vi "Select ECUMC Item.vi"(6 "NIVS.System Definition Root":refnum<k24>, 8 "error in (no error)":errorcluster, 9 "Item Type":T1=enum."Measurement", 11 "Link In":T2) -> (0 "error out":errorcluster, 1 "Canceled?":bool, 3 "Link Out":T2)   [LabVIEW 2011]
uses:
  <vilib>/ECUMC/NIVS/Support Files.llb/Comment Property.ctl
  <vilib>/ECUMC/NIVS/Support Files.llb/Address Property.ctl
  <vilib>/ECUMC/NIVS/Support Files.llb/Extension Property.ctl
  <vilib>/ECUMC/NIVS/Support Files.llb/Unit Property.ctl
  NationalInstruments.VeriStand.SystemStorage
  Controls/ECUMC Item.ctl
  <vilib>/ECUMC/NIVS/Support Files.llb/Item Type.ctl
  <vilib>/ECUMC/NIVS/Support Files.llb/Get Single Char Properties (TCP).vi
  <vilib>/ECUMC/NIVS/Support Files.llb/Get Single Meas Properties (TCP).vi
  <userlib>/_OpenG.lib/array/array.llb/Filter 1D Array__ogtk.vi
  <userlib>/_OpenG.lib/array/array.llb/Filter 1D Array with Scalar (String)__ogtk.vi
  <userlib>/_OpenG.lib/string/string.llb/String to 1D Array__ogtk.vi
  <vilib>/dlg_ctls.llb/Space Constant.vi
  NationalInstruments.VeriStand.SystemDefinitionAPI
  <vilib>/ECUMC/NIVS/Support Files.llb/XCP and CCP Master Custom Device.lvlib
  <vilib>/ECUMC/NIVS/XCPCCP Add-On Execution API.lvlib
panel:
  in  "Target":u16(ring) items=["FirstController"]
  in  "Cancel":bool
  in  "OK":bool
  out "Unit":T3
  out "Extension":T4
  out "Address":T5 format="%x"
  out "Comment":T6
  in  "Show results:":enum32{"Radio Selection 2", "Radio Selection 1"}(radio)
  in  "CaseSens":bool
  in  "Search":string
  in  "ItemList":i32(listbox) caption="Available Items in Database"
  in  "CD":u16(ring) caption="Custom Device" items=["XCP and CCP Master"]
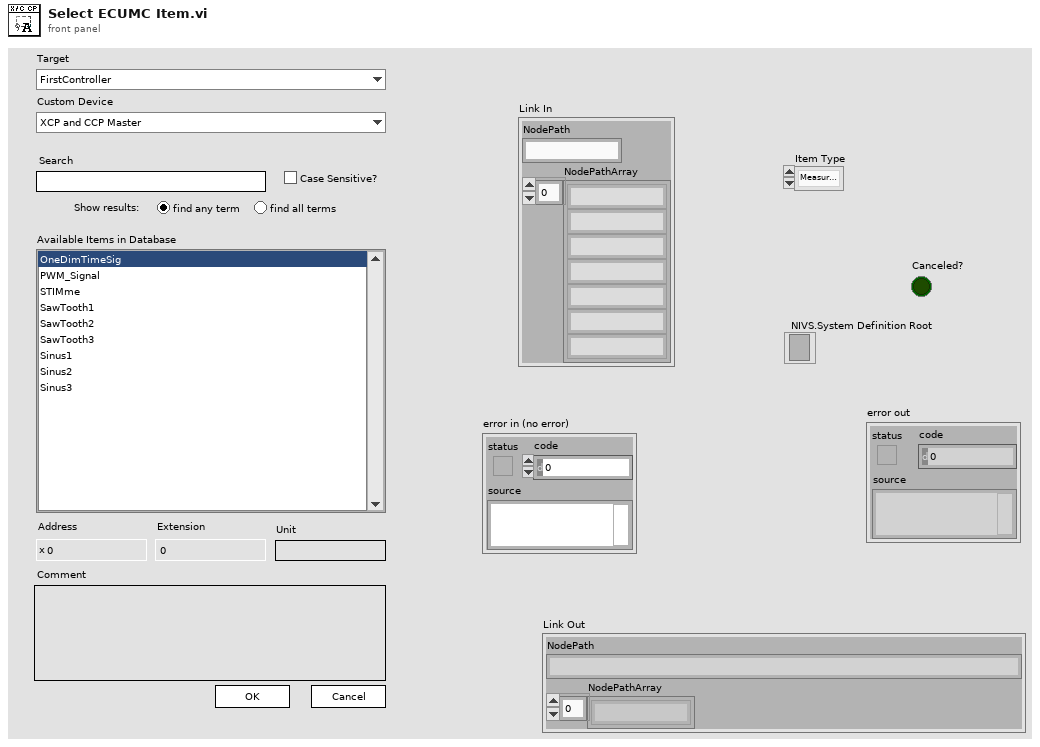
[diagram p1: front panel]
types:
  T1 = typedef "XCP and CCP Master Custom Device.lvlib/Item Type.ctl" = enum16{"Scalar Characteristic", "Curve Characteristic", "Field Characteristic", "Measurement"}
  T2 = typedef "ECUMC Item.ctl" = cluster{"NodePath":string, "NodePathArray":string[]}
  T3 = typedef "XCP and CCP Master Custom Device.lvlib/Unit Property.ctl" = string
  T4 = typedef "XCP and CCP Master Custom Device.lvlib/Extension Property.ctl" = u8
  T5 = typedef "XCP and CCP Master Custom Device.lvlib/Address Property.ctl" = u32
  T6 = typedef "XCP and CCP Master Custom Device.lvlib/Comment Property.ctl" = string
  T7 = typedef "XCP and CCP Master Custom Device.lvlib/Item Properties.ctl" = cluster{"Common":cluster{"Address":T5, "Extension":T4, "Data Type":T8, "Byte Order":T9, "Maximum":T10, "Minimum":T11, "Read Only?":T12, "Unit":T3, "Comment":T6}, "Char Specific":cluster{"X Dimension":T13, "Y Dimension":T14, "char x axis":dbl[], "char y axis":dbl[], "char sizes":u32[]}, "Meas Specific":cluster{"Virtual?":T15}}
  T8 = typedef "XCP and CCP Master Custom Device.lvlib/Data Type Property.ctl" = enum16{"UBYTE", "SBYTE", "UWORD", "SWORD", "ULONG", "SLONG", "FLOAT32_IEEE", "FLOAT64_IEEE"}
  T9 = typedef "XCP and CCP Master Custom Device.lvlib/Byte Order Property.ctl" = enum16{"Intel", "Motorola"}
  T10 = typedef "XCP and CCP Master Custom Device.lvlib/Maximum Property.ctl" = dbl
  T11 = typedef "XCP and CCP Master Custom Device.lvlib/Minimum Property.ctl" = dbl
  T12 = typedef "XCP and CCP Master Custom Device.lvlib/Read Only Property.ctl" = bool
  T13 = typedef "XCP and CCP Master Custom Device.lvlib/X Dimension Property.ctl" = u32
  T14 = typedef "XCP and CCP Master Custom Device.lvlib/Y Dimension Property.ctl" = u32
  T15 = typedef "XCP and CCP Master Custom Device.lvlib/Is Virtual Property.ctl" = bool
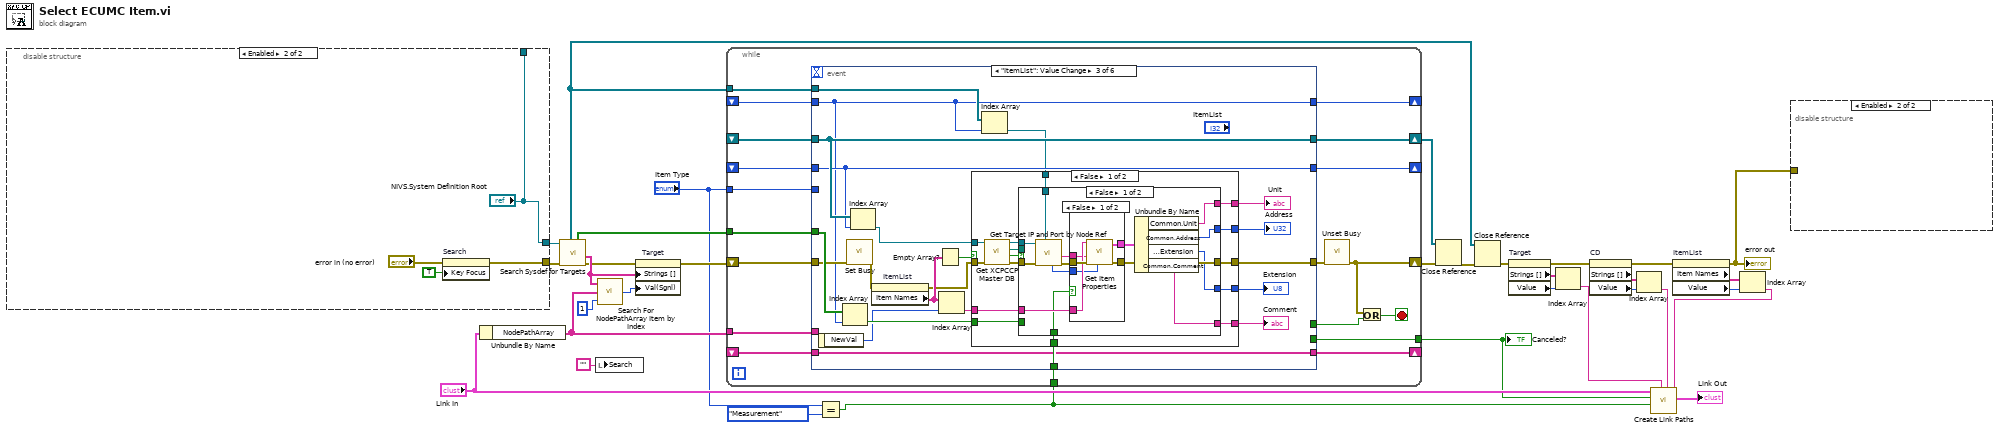
[diagram p0: block diagram]
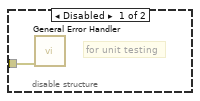
[diagram p2: hidden frame]
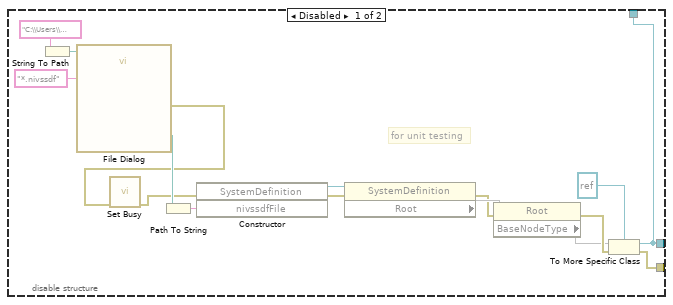
[diagram p3: hidden frame]
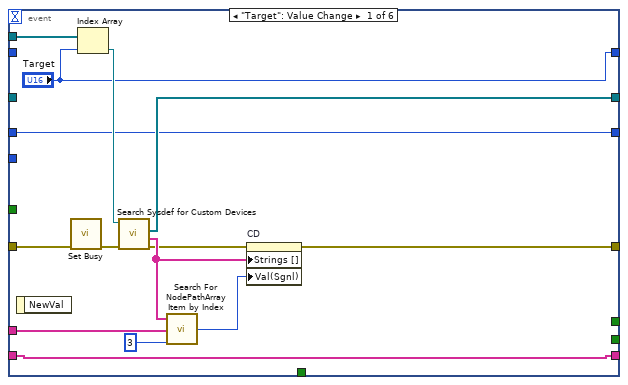
[diagram p4: hidden frame]
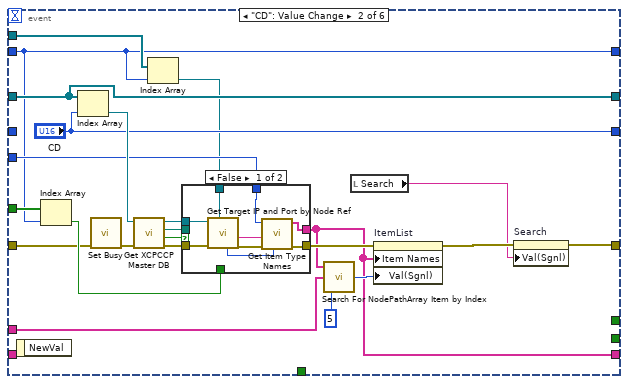
[diagram p5: hidden frame]
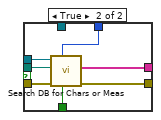
[diagram p6: hidden frame]
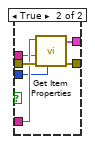
[diagram p7: hidden frame]
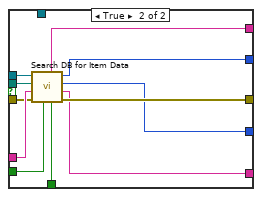
[diagram p8: hidden frame]
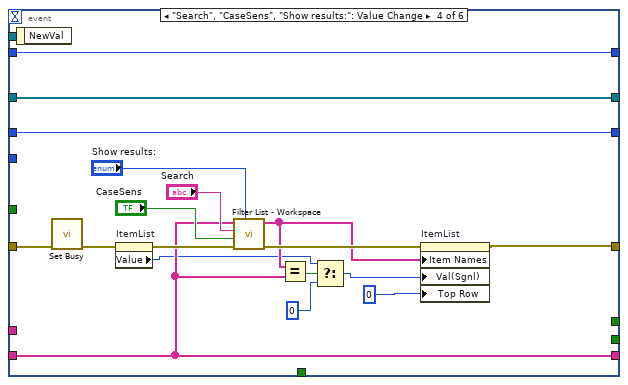
[diagram p10: hidden frame]
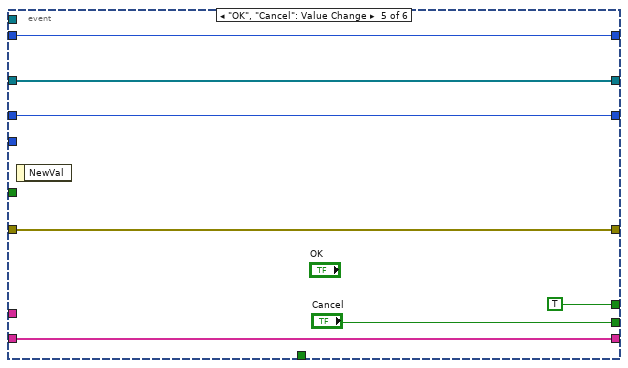
[diagram p11: hidden frame]
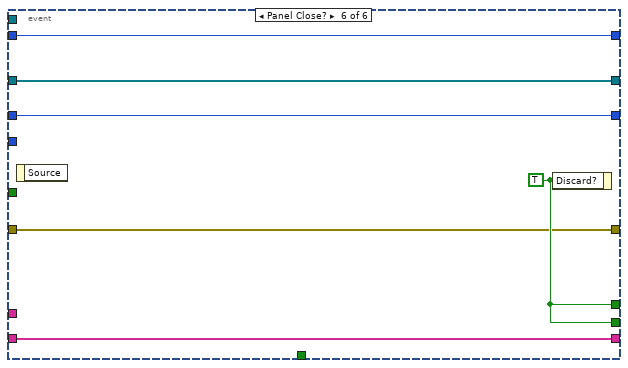
[diagram p12: hidden frame]
diagram:
  n1 = disable-structure shown="Enabled" {
    disable-tunnel: [w34 "NIVS.System Definition Root"] -> w32
    disable-tunnel: [w41 w50] -> w21
    disable-tunnel: [w34 "NIVS.System Definition Root"] -> _
    frame Disabled {
      # "for unit testing"
      n2 = String To Path(string="C:\\Users\\Public\\Documents\\National Instruments\\NI VeriStand 2010\\Projects") -> (path=w37:path)
      n3 = call "File Dialog"("start path"=w37, "pattern (all files)"="*.nivssdf") -> ("selected path"=w48:path, "error out"=w35:errorcluster)  [unwired: 10 in, 2 out]
      n4 = call <vilib>:"Set Busy.vi"("error in (no error)"=w35) -> ("error out"=w36:errorcluster)  [unwired: 9 in, 1 out]
      n5 = Path To String(path=w48) -> (string=w47:string)
      n6 = constructor class="SystemDefinition"(error in=w36, "nivssdfFile"=w47) -> (reference out=w45:refnum<k24>, error out=w46:errorcluster)  [unwired: 2 in, 2 out]
      n7 = property class="SystemDefinition"(reference=w45, error in=w46) -> (error out=w43:errorcluster, "Root"=w44)  [unwired: 1 out]
      n8 = property class="Root"(reference=w44, error in=w43) -> (error out=w42:errorcluster, "BaseNodeType"=w40)  [unwired: 1 out]
      n9 = To More Specific Class(target class=refnum<k24> refnum, reference=w40, error in=w42) -> (specific class reference=w34:refnum<k24>, error out=w41:errorcluster)
    }
    frame Enabled {
      n10 = property on="Search" class="Str"(error in="error in (no error)", "Key Focus"=TRUE) -> (error out=w50:errorcluster)  [unwired: 1 in, 1 out]
    }
  }
  n11 = Unbundle By Name("Link In") -> ("NodePathArray"=w27:string[])
  n12 = call "Search Sysdef for Targets.vi"("error in (no error)"=w21, "NIVS.System Definition Root"=w32) -> ("error out"=w22:errorcluster, "Target Names"=w29:string[], "Windows?"=w31:bool[], "Target Nodes"=w23:refnum<k24>[])  [unwired: 5 in, 1 out]
  n13 = local write "Search"("") -> ()
  n14 = call "Search For NodePathArray Item by Index.vi"("index of NodePathArray"=1 ("index"), "NodePathArray"=w27, "Items to search"=w29) -> ("result"=w28:i32)
  n15 = property on="Target" class="Ring (strict)"(error in=w22, "Strings []"=w29, "Val(Sgnl)"=w28) -> (error out=w5:errorcluster)  [unwired: 1 in, 1 out]
  n16 = Equal?(x="Item Type", y=Item_Type."Measurement") -> (x = y?=w2:bool)
  n17 = while {
    shift-right: [w54] -> w26
    shift-left: w5 -> [w72]
    tunnel: w31 -> [w70]
    tunnel: w27 -> [w69]
    tunnel: w23 -> [w68]
    tunnel: [w66] -> w19
    shift-right: [w65] -> w25
    shift-left: _ -> [w64]
    shift-right: [w63] -> _
    shift-left: _ -> [w62]
    shift-right: [w61] -> _
    shift-left: _ -> [w60]
    tunnel: "Item Type" -> [w59]
    tunnel: w2 -> [w58]
    shift-right: [w57] -> _
    shift-left: _ -> [w56]
    stop <- w71 stop-if-true
    n18 = event shown="[2] \"ItemList\": Value Change" {
      selector: _ -> [_ _ _ _ _ _]
      dyn-events: _ -> [_ _ _ _ _ _]
      timeout: _ -> [_ _ _ _ _ _]
      tunnel: w72 -> [w79 w101 w141 w203 w225 w226]
      tunnel: w70 -> [_ w103 w144 _ _ _]
      tunnel: w69 -> [w82 w106 _ _ _ _]
      tunnel: w68 -> [w86 w89 w137 _ _ _]
      tunnel: [_ _ _ _ TRUE w230] -> w67
      tunnel: [w73 w90 w126 w201 w225 w226] -> w55
      tunnel: [_ _ _ _ "Cancel" w230] -> w66
      tunnel: w62 -> [_ w88 w136 w212 w220 w227]
      tunnel: [w84 w99 w147 w213 w222 w228] -> w65
      tunnel: w64 -> [_ w99 w147 w213 w222 w228]
      tunnel: ["Target" w88 w136 w212 w220 w227] -> w63
      tunnel: [w75 "CD" w146 w214 w221 w229] -> w61
      tunnel: w60 -> [w75 _ w146 w214 w221 w229]
      tunnel: w59 -> [_ w96 _ _ _ _]
      tunnel: w58 -> [_ _ w142 _ _ _]
      tunnel: [w74 w95 w140 w209 w219 w231] -> w57
      tunnel: w56 -> [w74 _ w140 w209 w219 w231]
      event "Target": Value Change {
        n19 = event-data() -> ()  [unwired: 1 in, 1 out]
        n20 = call <vilib>:"Set Busy.vi"("error in (no error)"=w79) -> ("error out"=w78:errorcluster)  [unwired: 9 in, 1 out]
        n21 = Index Array(array=w86, index="Target") -> (element=w85:refnum<k24>)
        n22 = call "Search Sysdef for Custom Devices.vi"("error in (no error)"=w78, "Target Node"=w85) -> ("error out"=w77:errorcluster, "Custom Device Names"=w83:string[], "Custom Device Nodes"=w84:refnum<k24>[])  [unwired: 6 in, 1 out]
        n23 = call "Search For NodePathArray Item by Index.vi"("index of NodePathArray"=3 ("index"), "NodePathArray"=w82, "Items to search"=w83) -> ("result"=w80:i32)
        n24 = property on="CD" class="Ring (strict)"(error in=w77, "Strings []"=w83, "Val(Sgnl)"=w80) -> (error out=w73:errorcluster)  [unwired: 1 in, 1 out]
      }
      event "CD": Value Change {
        n25 = event-data() -> ()  [unwired: 1 in, 1 out]
        n26 = Index Array(array=w103, index=w88) -> (element=w102:bool)
        n27 = Index Array(array=w99, index="CD") -> (element=w109:refnum<k24>)
        n28 = call <vilib>:"Set Busy.vi"("error in (no error)"=w101) -> ("error out"=w100:errorcluster)  [unwired: 9 in, 1 out]
        n29 = call "Get XCPCCP Master DB.vi"("error in (no error)"=w100, "Custom Device Node in"=w109) -> ("error out"=w108:errorcluster, "file or folder exists?"=w92:bool, "DB Path"=w91:path, "Custom Device Node out"=w107:refnum<k24>)  [unwired: 6 in]
        n30 = Index Array(array=w89, index=w88) -> (element=w87:refnum<k24>)
        n31 = case shown="False" w92 {
          tunnel: w108 -> [w115 w125]
          tunnel: w91 -> [_ w120]
          tunnel: w107 -> [w114 w123]
          tunnel: [w117 w121] -> w95
          tunnel: [w118 w124] -> w104
          tunnel: w96 -> [w116 w122]
          tunnel: w102 -> [_ w119]
          tunnel: w87 -> [w113 _]
          frame False {
            n32 = call "Get Target IP and Port by Node Ref.vi"("Target Node In"=w113, "error in (no error)"=w115, "Custom Device Node in"=w114) -> ("error out"=w111:errorcluster, "IP"=w110:string, "Port"=w112:u16)  [unwired: 6 in]
            n33 = call <vilib>:"Get Item Type Names.vi"("Port"=w112, "error in (no error)"=w111, "IP or DNS Name"=w110, "Item Type"=w116) -> ("error out"=w118:errorcluster, "Names"=w117:string[])  [unwired: 6 in]
          }
          frame True {
            n34 = call "Search DB for Chars or Meas.vi"("Windows? (F)"=w119, "Item Type"=w122, "error in (no error)"=w125, "DB Path"=w120, "Custom Device Node in"=w123) -> ("error out"=w124:errorcluster, "Chans"=w121:string[])  [unwired: 4 in, 1 out]
          }
        }
        n35 = call "Search For NodePathArray Item by Index.vi"("index of NodePathArray"=5, "NodePathArray"=w106, "Items to search"=w95) -> ("result"=w98:i32)
        n36 = local read "Search"() -> (w93:string)
        n37 = property on="ItemList" class="LstBox (strict)"(error in=w104, "Item Names"=w95, "Val(Sgnl)"=w98) -> (error out=w94:errorcluster)  [unwired: 1 in, 1 out]
        n38 = property on="Search" class="Str"(error in=w94, "Val(Sgnl)"=w93) -> (error out=w90:errorcluster)  [unwired: 1 in, 1 out]
      }
      event "ItemList": Value Change {
        n39 = event-data() -> ("NewVal"=w139:i32)  [unwired: 1 in]
        n40 = Index Array(array=w144, index=w136) -> (element=w143:bool)
        n41 = call <vilib>:"Set Busy.vi"("error in (no error)"=w141) -> ("error out"=w130:errorcluster)  [unwired: 9 in, 1 out]
        n42 = Index Array(array=w147, index=w146) -> (element=w145:refnum<k24>)
        n43 = property on="ItemList" class="LstBox (strict)"(error in=w130) -> (error out=w128:errorcluster, "Item Names"=w129:string[])  [unwired: 1 in, 1 out]
        n44 = Empty Array?(array=w129) -> (empty?=w127:bool)
        n45 = Index Array(array=w129, index=w139) -> (element=w138:string)
        n46 = Index Array(array=w137, index=w136) -> (element=w135:refnum<k24>)
        n47 = case shown="False" w127 {
          tunnel: w145 -> [w162 _]
          tunnel: w143 -> [w160 _]
          tunnel: w142 -> [w157 _]
          tunnel: [w156 w200] -> w126
          tunnel: w138 -> [w155 _]
          tunnel: w135 -> [w154 _]
          tunnel: [w153 _] -> w134
          tunnel: [w152 _] -> w133
          tunnel: [w151 _] -> w132
          tunnel: [w150 _] -> w131
          tunnel: w128 -> [w149 w200]
          frame False {
            n48 = call "Get XCPCCP Master DB.vi"("error in (no error)"=w149, "Custom Device Node in"=w162) -> ("error out"=w148:errorcluster, "file or folder exists?"=w161:bool, "DB Path"=w158:path, "Custom Device Node out"=w159:refnum<k24>)  [unwired: 6 in]
            n49 = case shown="False" w161 {
              tunnel: w160 -> [_ w199]
              tunnel: w159 -> [w173 w198]
              tunnel: w158 -> [_ w197]
              tunnel: w148 -> [w175 w193]
              tunnel: w157 -> [w168 w196]
              tunnel: [w169 w195] -> w156
              tunnel: w155 -> [w176 w194]
              tunnel: w154 -> [w172 _]
              tunnel: [w163 w192] -> w153
              tunnel: [w164 w191] -> w152
              tunnel: [w165 w190] -> w151
              tunnel: [w166 w189] -> w150
              frame False {
                n50 = call "Get Target IP and Port by Node Ref.vi"("Target Node In"=w172, "error in (no error)"=w175, "Custom Device Node in"=w173) -> ("error out"=w174:errorcluster, "IP"=w170:string, "Port"=w171:u16)  [unwired: 6 in]
                n51 = case shown="False" w168 {
                  tunnel: w174 -> [w182 w188]
                  tunnel: w176 -> [w181 w187]
                  tunnel: w171 -> [w180 w186]
                  tunnel: w170 -> [w179 w185]
                  tunnel: [w178 w184] -> w169
                  tunnel: [w177 w183] -> w167
                  frame False {
                    n52 = call-poly <vilib>:"Get Item Properties.vi"("Port"=w180, "error in (no error)"=w182, "IP or DNS Name"=w179, "Characteristic"=w181) -> ("error out"=w178:errorcluster, "Properties"=w177:T7)  [unwired: 6 in]
                  }
                  frame True {
                    n53 = call-poly <vilib>:"Get Item Properties.vi"("Port"=w186, "error in (no error)"=w188, "IP or DNS Name"=w185, "Measurement"=w187) -> ("error out"=w184:errorcluster, "Properties"=w183:T7)  [unwired: 6 in]
                  }
                }
                n54 = Unbundle By Name(w167) -> ("Common.Unit"=w166:T3, "Common.Address"=w165:T5, "Common.Extension"=w164:T4, "Common.Comment"=w163:T6)
              }
              frame True {
                n55 = call "Search DB for Item Data.vi"("Measurement? (F)"=w196, "Windows? (F)"=w199, "error in (no error)"=w193, "Item Name"=w194, "DB Path"=w197, "Custom Device Node in"=w198) -> ("error out"=w195:errorcluster, "Comment"=w192:string, "Extension"=w191:u8, "Address"=w190:u32, "Unit"=w189:string)  [unwired: 1 in]
              }
            }
          }
          frame True {
          }
        }
        "Address" <- w132
        "Extension" <- w133
        "Unit" <- w131
        "Comment" <- w134
      }
      event "Search", "CaseSens", "Show results:": Value Change {
        n56 = event-data() -> ()  [unwired: 1 in, 1 out]
        n57 = call <vilib>:"Set Busy.vi"("error in (no error)"=w203) -> ("error out"=w202:errorcluster)  [unwired: 9 in, 1 out]
        n58 = property on="ItemList" class="LstBox (strict)"(error in=w202) -> (error out=w211:errorcluster, "Value"=w205:i32)  [unwired: 1 in, 1 out]
        n59 = call "Filter List - Workspace.vi"("Filter results:"="Show results:", "error in (no error)"=w211, "CaseSens"="CaseSens", "Filter String"="Search", "names list in"=w209) -> ("error out"=w215:errorcluster, "names list out"=w210:string[])  [unwired: 4 in]
        n60 = Equal?(x=w210, y=w209) -> (x = y?=w208:bool)
        n61 = Select(t=w205, s=w208, f=0 ("Top Row")) -> (s? t:f=w204:i32)
        n62 = property on="ItemList" class="LstBox (strict)"(error in=w215, "Item Names"=w210, "Val(Sgnl)"=w204, "Top Row"=0) -> (error out=w201:errorcluster)  [unwired: 1 in, 1 out]
      }
      event "OK", "Cancel": Value Change {
        n63 = event-data() -> ()  [unwired: 1 in, 1 out]
      }
      event Panel Close? {
        w230 = TRUE ("Discard?")
        n64 = event-data() -> ()  [unwired: 1 in, 1 out]
        n65 = event-data("Discard?"=w230) -> ()  [unwired: 1 in, 1 out]
      }
    }
    n66 = call <vilib>:"Unset Busy.vi"("error in (no error)"=w55) -> ("error out"=w54:errorcluster)  [unwired: 10 in]
    n67 = Or(x=w54, y=w67) -> (x .or. y?=w71:bool)
  }
  "Canceled?" <- w19
  n68 = Close Reference(reference=w25, error in (no error)=w26) -> (error out=w24:errorcluster)
  n69 = Close Reference(reference=w23, error in (no error)=w24) -> (error out=w9:errorcluster)
  n70 = property on="Target" class="Ring (strict)"(error in=w9) -> (error out=w8:errorcluster, "Strings []"=w11:string[], "Value"=w10:u16)  [unwired: 1 in, 1 out]
  n71 = Index Array(array=w11, index=w10) -> (element=w7:string)
  n72 = property on="CD" class="Ring (strict)"(error in=w8) -> (error out=w12:errorcluster, "Strings []"=w14:string[], "Value"=w15:u16)  [unwired: 1 in, 1 out]
  n73 = Index Array(array=w14, index=w15) -> (element=w13:string)
  n74 = property on="ItemList" class="LstBox (strict)"(error in=w12) -> (error out=w1:errorcluster, "Item Names"=w18:string[], "Value"=w17:i32)  [unwired: 1 in, 1 out]
  "error out" <- w1
  n75 = Index Array(array=w18, index=w17) -> (element=w16:string)
  n76 = call "Create Link Paths.vi"("Item"=w16, "CD"=w13, "Target"=w7, "Measurement? (F)"=w2, "Canceled?"=w19, "Link In"="Link In") -> ("Link Out"=→"Link Out":T2)  [unwired: 5 in]
  n77 = disable-structure shown="Enabled" {
    disable-tunnel: w1 -> [w232 _]
    frame Disabled {
      # "for unit testing"
      n78 = call <vilib>:"General Error Handler.vi"("error in (no error)"=w232) -> ()  [unwired: 10 in, 5 out]
    }
    frame Enabled {
    }
  }
